vi "Create Channel Task.vi"(8 "error in":errorcluster, 11 "NI Digital Output in":refnum<class "NI Digital Output.lvclass">) -> (0 "error out":errorcluster, 3 "NI Digital Output out":refnum<class "NI Digital Output.lvclass">)   [LabVIEW 2023, in "HardwareAbstractionLayer_LVOOP.lvlib" / "NI Digital Output.lvclass"]
doc: "This VI Analog Output Physical Channel Based DAQmx Create Channel"
uses:
  NI Digital Output.lvclass
  NI Digital Output.lvclass/NI Digital Output.ctl
  <vilib>/DAQmx/create/channels.llb/DAQmx Create Channel (DO-Digital Output).vi
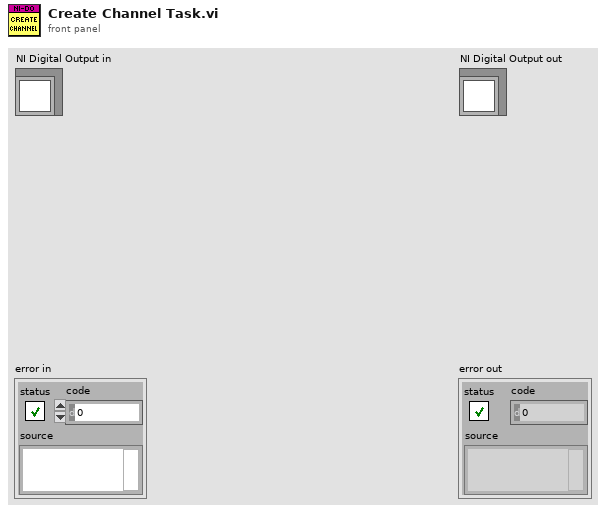
[diagram p1: front panel]
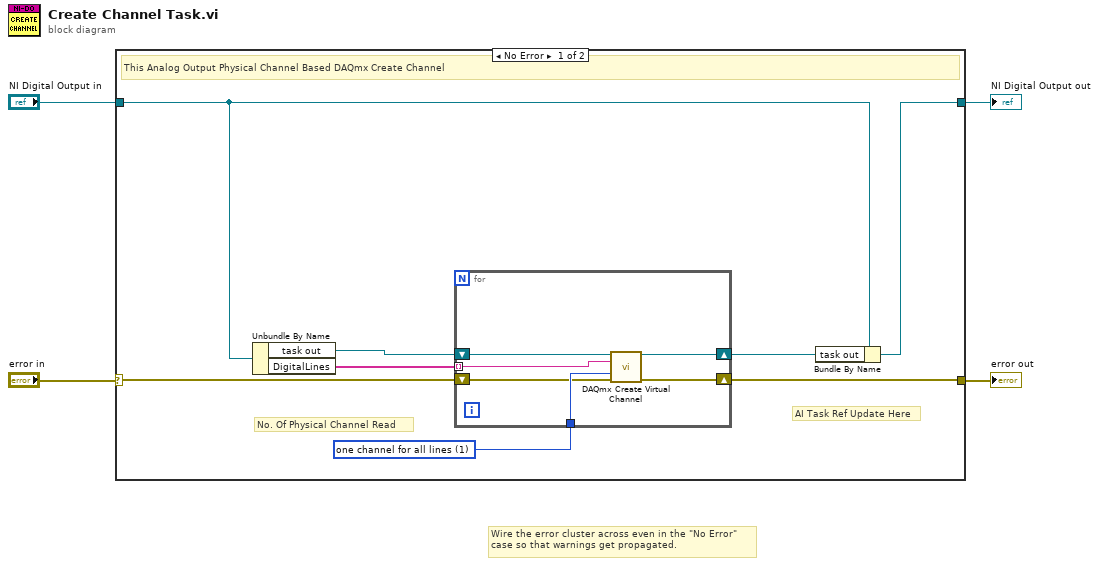
[diagram p0: block diagram]
diagram:
  # "Wire the error cluster across even in the \"No Error\"\ncase so that warnings get propagated."
  n1 = case shown="No Error" "error in" {
    selector: "error in" -> [w6 w20]
    tunnel: [w7 w20] -> w3
    tunnel: [w11 w19] -> w1
    tunnel: "NI Digital Output in" -> [w10 w19]
    frame No Error {
      w9 = 1 items=["one channel for each line", "one channel for all lines"] ("line grouping")
      # "AI Task Ref Update Here"
      # "No. Of Physical Channel Read"
      # "This Analog Output Physical Channel Based DAQmx Create Channel"
      n2 = Unbundle By Name(w10) -> ("task out"=w12:refnum<k21>, "DigitalLines"=w5:tag[])
      n3 = for {
        tunnel: w9 -> [w17]
        shift-right: [w16] -> w8
        shift-left: w12 -> [w18]
        shift-right: [w15] -> w7
        shift-left: w6 -> [w14]
        tunnel: w5 -> [w13] mode=indexing
        n4 = call-poly <vilib>:"DAQmx Create Virtual Channel.vi"("task in"=w18, "lines"=w13, "line grouping"=w17, "error in"=w14) -> ("task out"=w16:refnum<k21>, "error out"=w15:errorcluster)  [unwired: 10 in]
      }
      n5 = Bundle By Name(cluster=w10, "task out"=w8) -> (w11:refnum<class "NI Digital Output.lvclass">)
    }
    frame Error {
    }
  }
  "error out" <- w3
  "NI Digital Output out" <- w1
